vi "Color Picker Dialog.vi"(0 "Color In":u32(colorbox), 2 "parent":refnum<vi>, 7 "Coords":T1={"Horizontal"=-1, "Vertical"=-1}) -> (4 "Color Out":u32(colorbox), 8 "Canceled?":bool)   [LabVIEW 2020]
uses:
  <vilib>/Utility/miscctls.llb/LVPoint32TypeDef.ctl
panel:
  in  "Color Box":u32(colorbox) caption="Click to change color"
  in  "Cancel":bool
  in  "OK":bool
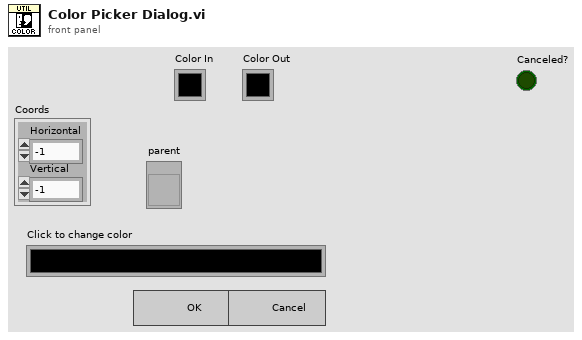
[diagram p1: front panel]
types:
  T1 = typedef "LVPoint32TypeDef.ctl" = cluster{"Horizontal":i32, "Vertical":i32}
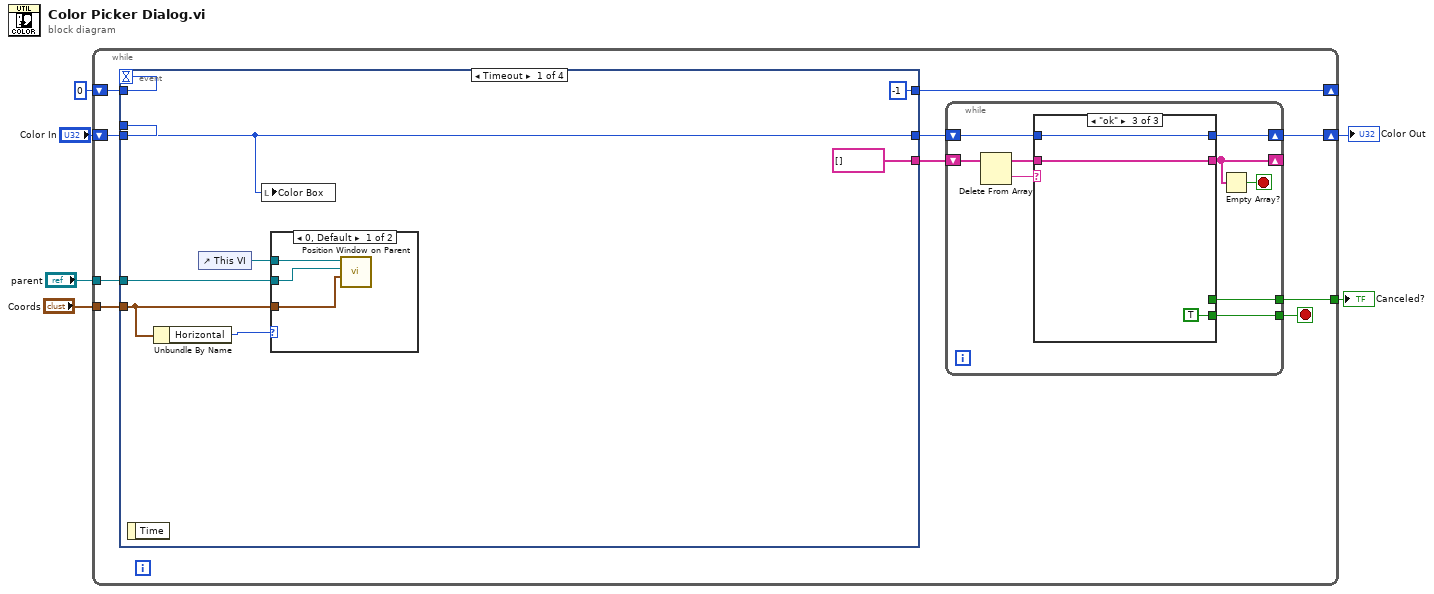
[diagram p0: block diagram]
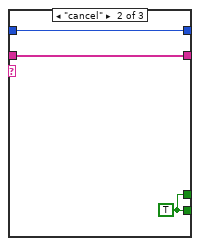
[diagram p3: hidden frame]
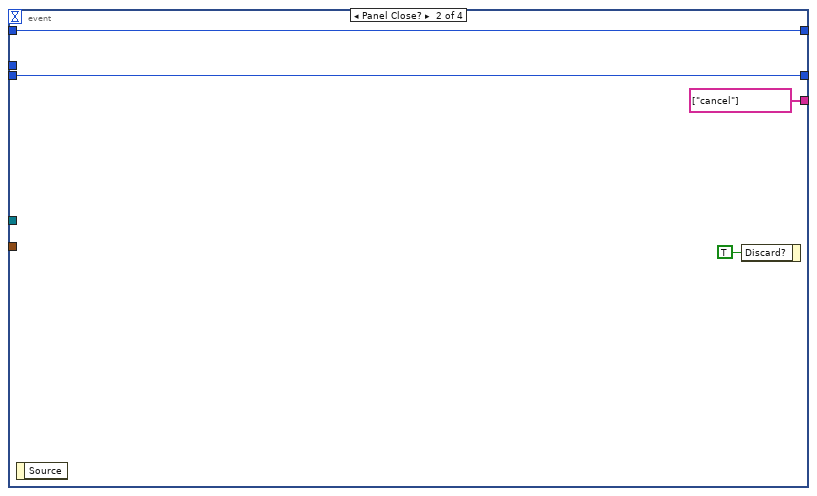
[diagram p5: hidden frame]
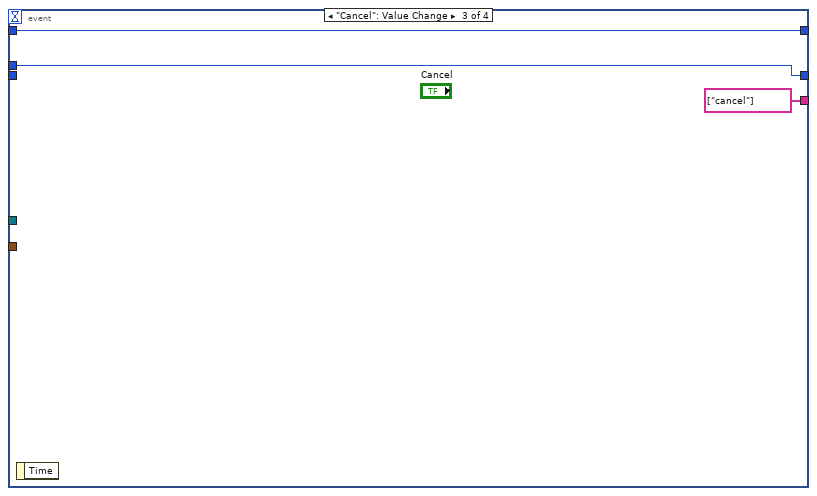
[diagram p6: hidden frame]
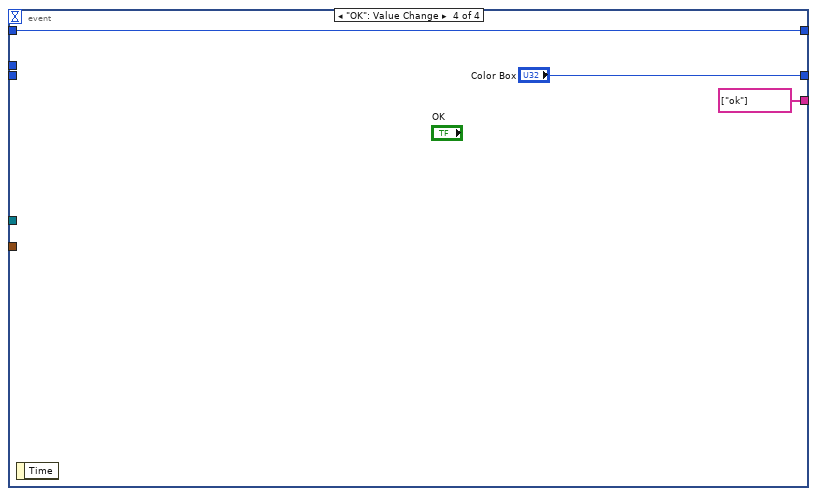
[diagram p7: hidden frame]
diagram:
  n1 = while {
    shift-right: [w16] -> _
    shift-left: 0 -> [w14]
    tunnel: [w9] -> w3
    shift-right: [w10] -> w4
    shift-left: "Color In" -> [w15]
    tunnel: "Coords" -> [w8]
    tunnel: "parent" -> [w7]
    stop <- w11 stop-if-true
    n2 = event shown="[0] Timeout" {
      selector: _ -> [_ _ _ _]
      dyn-events: _ -> [_ _ _ _]
      timeout: w14 -> [_ _ _ _]
      tunnel: [-1 w47 w49 w53] -> w16
      tunnel: w15 -> [w38 w46 _ _]
      tunnel: [w38 w46 w50 "Color Box"] -> w13
      tunnel: w15 -> [_ _ w50 _]
      tunnel: w14 -> [_ w47 w49 w53]
      tunnel: [string[] [] string[] ["cancel"] string[] ["cancel"] string[] ["ok"]] -> w12
      tunnel: w8 -> [w35 _ _ _]
      tunnel: w7 -> [w34 _ _ _]
      event Timeout {
        n3 = event-data() -> ()  [unwired: 1 in, 1 out]
        n4 = Unbundle By Name(w35) -> ("Horizontal"=w36:i32)
        n5 = control-ref of="This VI"() -> (w37:refnum<vi>)
        n6 = local write "Color Box"(w38) -> ()
        n7 = case shown="0, Default" w36 {
          tunnel: w37 -> [w43 _]
          tunnel: w35 -> [w42 _]
          tunnel: w34 -> [w41 _]
          frame 0, Default {
            n8 = call "Position Window on Parent.vi"("Offset"=w42, "Parent VI"=w41, "VI in"=w43) -> ()  [unwired: 7 in, 2 out]
          }
          frame -1 {
          }
        }
      }
      event Panel Close? {
        n9 = event-data() -> ()  [unwired: 1 in, 1 out]
        n10 = event-data("Discard?"=TRUE) -> ()  [unwired: 1 in, 1 out]
      }
      event "Cancel": Value Change {
        n11 = event-data() -> ()  [unwired: 1 in, 1 out]
      }
      event "OK": Value Change {
        n12 = event-data() -> ()  [unwired: 1 in, 1 out]
      }
    }
    n13 = while {
      shift-right: [w22] -> _
      shift-left: w12 -> [w25]
      shift-right: [w19] -> w10
      shift-left: w13 -> [w20]
      tunnel: [w18] -> w11
      tunnel: [w17] -> w9
      stop <- w21 stop-if-true
      n14 = Delete From Array(array=w25) -> (deleted portion=w23:string, array with subset deleted=w24:string[])  [unwired: 2 in]
      n15 = case shown="\"ok\"" w23 {
        tunnel: w24 -> [w27 w30 w33]
        tunnel: [w27 w30 w33] -> w22
        tunnel: w20 -> [w26 w29 w32]
        tunnel: [w26 w29 w32] -> w19
        tunnel: [_ w28 TRUE] -> w18
        tunnel: [_ w28 _] -> w17
        frame "", Default {
        }
        frame "cancel" {
          w28 = TRUE
        }
        frame "ok" {
        }
      }
      n16 = Empty Array?(array=w22) -> (empty?=w21:bool)
    }
  }
  "Color Out" <- w4
  "Canceled?" <- w3
